vi "s_to_us_DBL.vi"(4 "time in":dbl caption="time in [s]" format="%#.6f") -> (1 "time out":dbl caption="time out [µs]" format="%#.6f")   [LabVIEW 2017, in "GPTiming.lvlib"]
doc: "Multiplies <B>time in</B> by 1,000,000 to convert it from seconds to microseconds.\n\nEven though its functionality is really simple this function is valuable as it documents your code much better than a raw multiplication by 1,000,000.\n\nThis VI is inlined.\n\nSteen Schmidt\nGPower\n9/12 2013"
uses:
  GPTiming.lvlib
panel:
  # "Copyright © 2013\nGPower\nSee enclosed license file for terms and conditions"
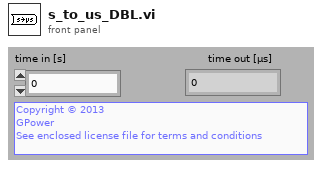
[diagram p1: front panel]
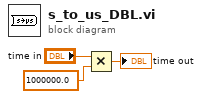
[diagram p0: block diagram]
diagram:
  n1 = Multiply(x="time in", y=1000000.0) -> (x*y=→"time out":dbl)
